vi "STL_Initialisation.vi"(8 "error in (no error)":errorcluster, 10 "Color":u32(colorbox)=1244928, 11 "Model File":path) -> (0 "error out":errorcluster, 3 "New Mesh Refnum":refnum<vi>)   [LabVIEW 2015]
uses:
  <vilib>/picture/3D Picture Control/NI_Old 3D Toolkit.lvlib
  <vilib>/picture/3D Picture Control/NI_3D Picture Control.lvlib
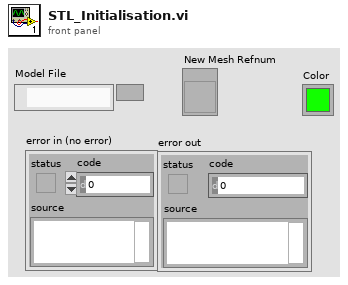
[diagram p1: front panel]
types:
  T1 = typedef "NI_3D Picture Control.lvlib/NI_Old 3D Toolkit.lvlib/model.ctl" = cluster{"VertexList":T2[], "FaceList":cluster{"v1":i32, "v2":i32, "v3":i32}[], "NormalList":T2[], "Mode":T3}
  T2 = typedef "NI_3D Picture Control.lvlib/NI_Old 3D Toolkit.lvlib/point3f.ctl" = cluster{"x":sgl, "y":sgl, "z":sgl}
  T3 = typedef "NI_3D Picture Control.lvlib/NI_Old 3D Toolkit.lvlib/VertexMode.ctl" = enum16{"GL_POINTS", "GL_LINES", "GL_LINE_LOOP", "GL_LINE_STRIP", "GL_TRIANGLES", "GL_TRIANGLE_STRIP", "GL_TRIANGLE_FAN", "GL_QUADS", "GL_QUAD_STRIP", "GL_POLYGON"}
  T4 = enum16{"Points", "Lines", "Line Strip", "Line Loop", "Triangles", "Triangle Strip", "Triangle Fan", "Quads", "Quad Strip", "Polygon"}
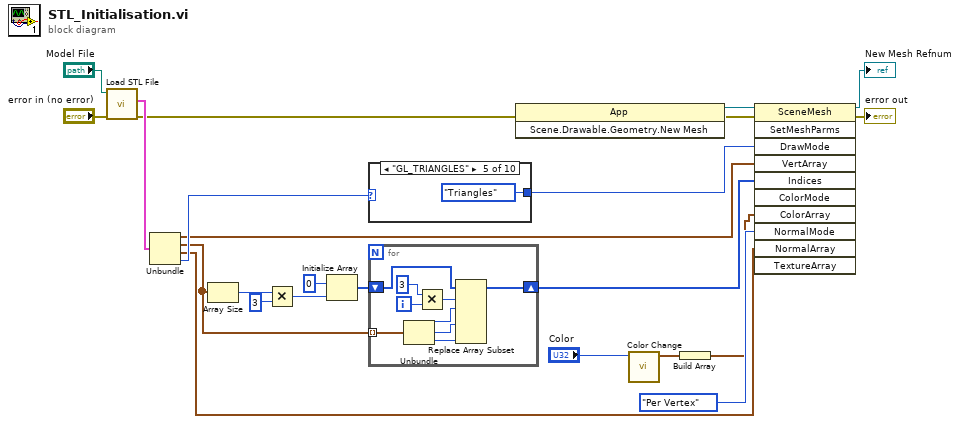
[diagram p0: block diagram]
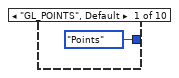
[diagram p2: hidden frame]
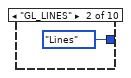
[diagram p3: hidden frame]
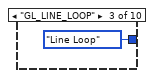
[diagram p4: hidden frame]
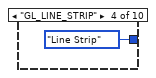
[diagram p5: hidden frame]
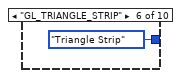
[diagram p6: hidden frame]
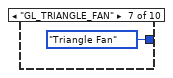
[diagram p7: hidden frame]
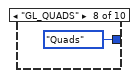
[diagram p8: hidden frame]
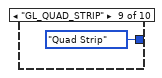
[diagram p9: hidden frame]
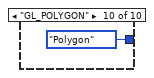
[diagram p10: hidden frame]
diagram:
  n1 = call <vilib>:"Load STL File.vi"("error in (no error)"="error in (no error)", "path to STL file"="Model File") -> ("error out"=w18:errorcluster, "Model Out"=w23:T1)  [unwired: 8 out]
  n2 = Unbundle(w23) -> ("VertexList"=w14:T2[], "FaceList"=w9:cluster{"v1":i32, "v2":i32, "v3":i32}[], "NormalList"=w13:T2[], "Mode"=w22:T3)
  n3 = Array Size(array=w9) -> (size(s)=w5:i32)
  n4 = Multiply(x=w5, y=3 ("x")) -> (x*y=w4:i32)
  n5 = Initialize Array(0 ("v3"), w4) -> (w8:i32[])
  n6 = case shown="\"GL_TRIANGLES\"" w22 {
    tunnel: [T4."Points" ("Draw Mode") T4."Lines" ("Draw Mode") T4."Line Loop" ("Draw Mode") T4."Line Strip" ("Draw Mode") T4."Triangles" ("Draw Mode") T4."Triangle Strip" ("Draw Mode") T4."Triangle Fan" ("Draw Mode") T4."Quads" ("Draw Mode") T4."Quad Strip" ("Draw Mode") T4."Polygon" ("Draw Mode")] -> w10
    frame "GL_POINTS", Default {
    }
    frame "GL_LINES" {
    }
    frame "GL_LINE_LOOP" {
    }
    frame "GL_LINE_STRIP" {
    }
    frame "GL_TRIANGLES" {
    }
    frame "GL_TRIANGLE_STRIP" {
    }
    frame "GL_TRIANGLE_FAN" {
    }
    frame "GL_QUADS" {
    }
    frame "GL_QUAD_STRIP" {
    }
    frame "GL_POLYGON" {
    }
  }
  n7 = for {
    tunnel: w9 -> [w42] mode=indexing
    shift-right: [w41] -> w11
    shift-left: w8 -> [w40]
    i -> [w36]
    n8 = Unbundle(w42) -> ("v1"=w39:i32, "v2"=w38:i32, "v3"=w37:i32)
    n9 = Multiply(x=3, y=w36) -> (x*y=w34:i32)
    n10 = Replace Array Subset(array=w40, new element #1=w39, index #1=w34, new element #2=w38, new element #3=w37) -> (w41:i32[])  [unwired: 2 in]
  }
  n11 = invoke class="App" method="Scene.Drawable.Geometry.New Mesh"(error in=w18) -> (error out=w17:errorcluster, "Scene.Geometry.New Mesh"=w21:refnum<vi>)  [unwired: 2 in, 1 out]
  n12 = call <vilib>:"Color Change.vi"("Color"="Color") -> ("RGBA"=w2:cluster{"R":sgl, "G":sgl, "B":sgl, "A":sgl})  [unwired: 10 in]
  n13 = Build Array(w2) -> (w1:cluster{"R":sgl, "G":sgl, "B":sgl, "A":sgl}[])
  n14 = invoke class="SceneMesh" method="SetMeshParms"(reference=w21, error in=w17, "DrawMode"=w10, "VertArray"=w14, "Indices"=w11, "ColorArray"=w1, "NormalMode"=enum16{"Overall", "Per Primitive", "Per Vertex"}."Per Vertex" ("Normal Binding Mode"), "NormalArray"=w13) -> (reference out=→"New Mesh Refnum":refnum<vi>, error out=→"error out":errorcluster)  [unwired: 3 in, 9 out]
